vi "Sequencer Pro.vi"(8 "error in (no error)":errorcluster) -> (0 "Error State":errorcluster)   [LabVIEW 2017]
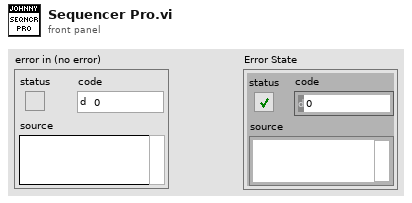
[diagram p1: front panel]
types:
  T1 = cluster{"Error State":errorcluster, "State_ndx":i32, "Timeout [s]":dbl}
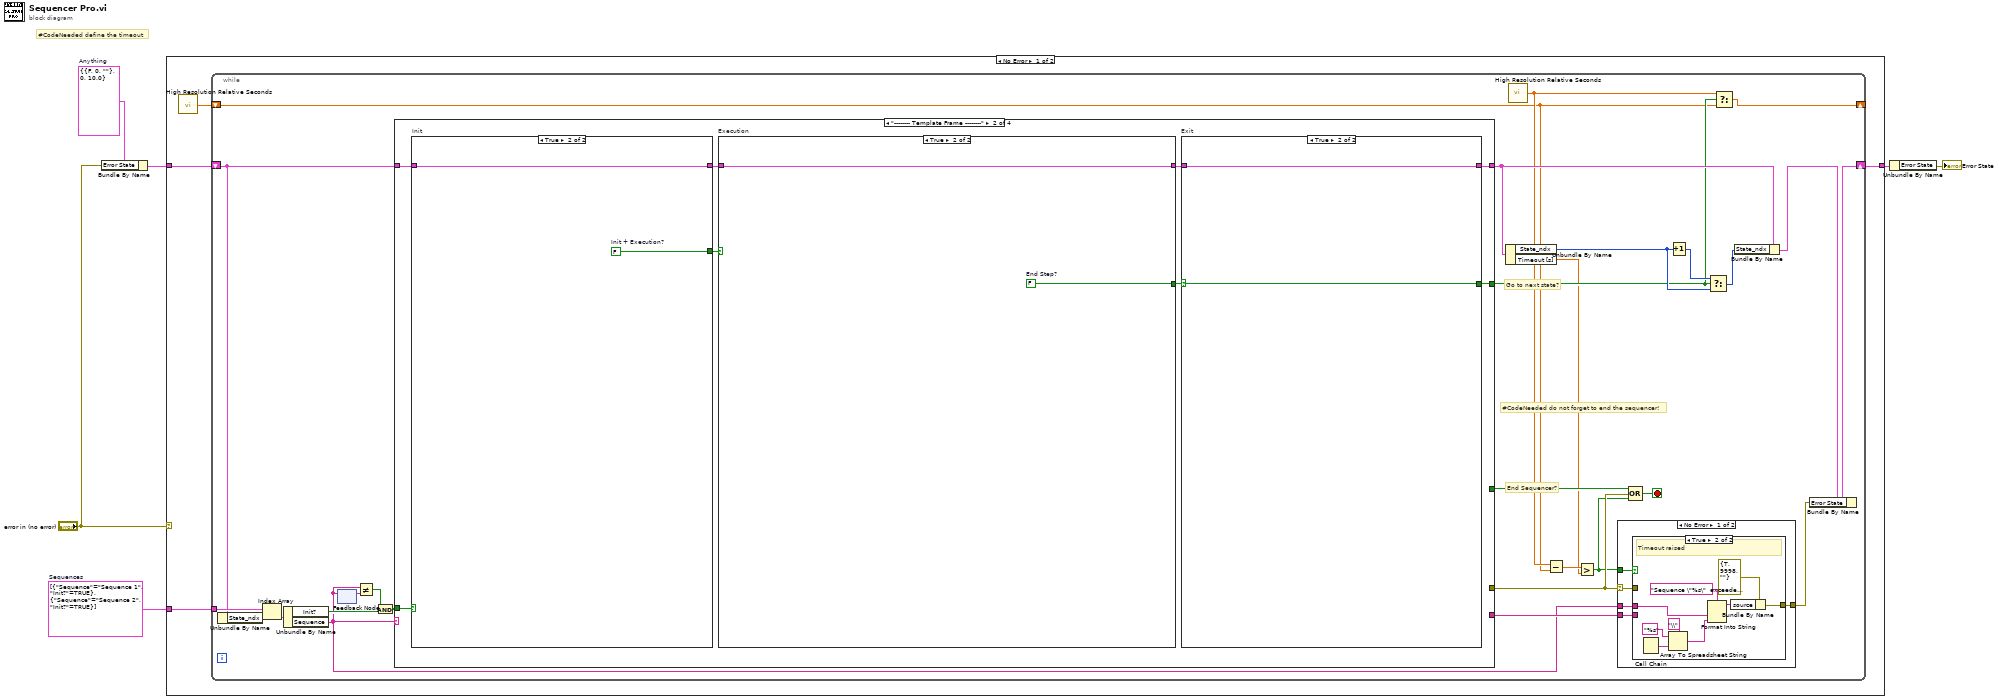
[diagram p0: block diagram]
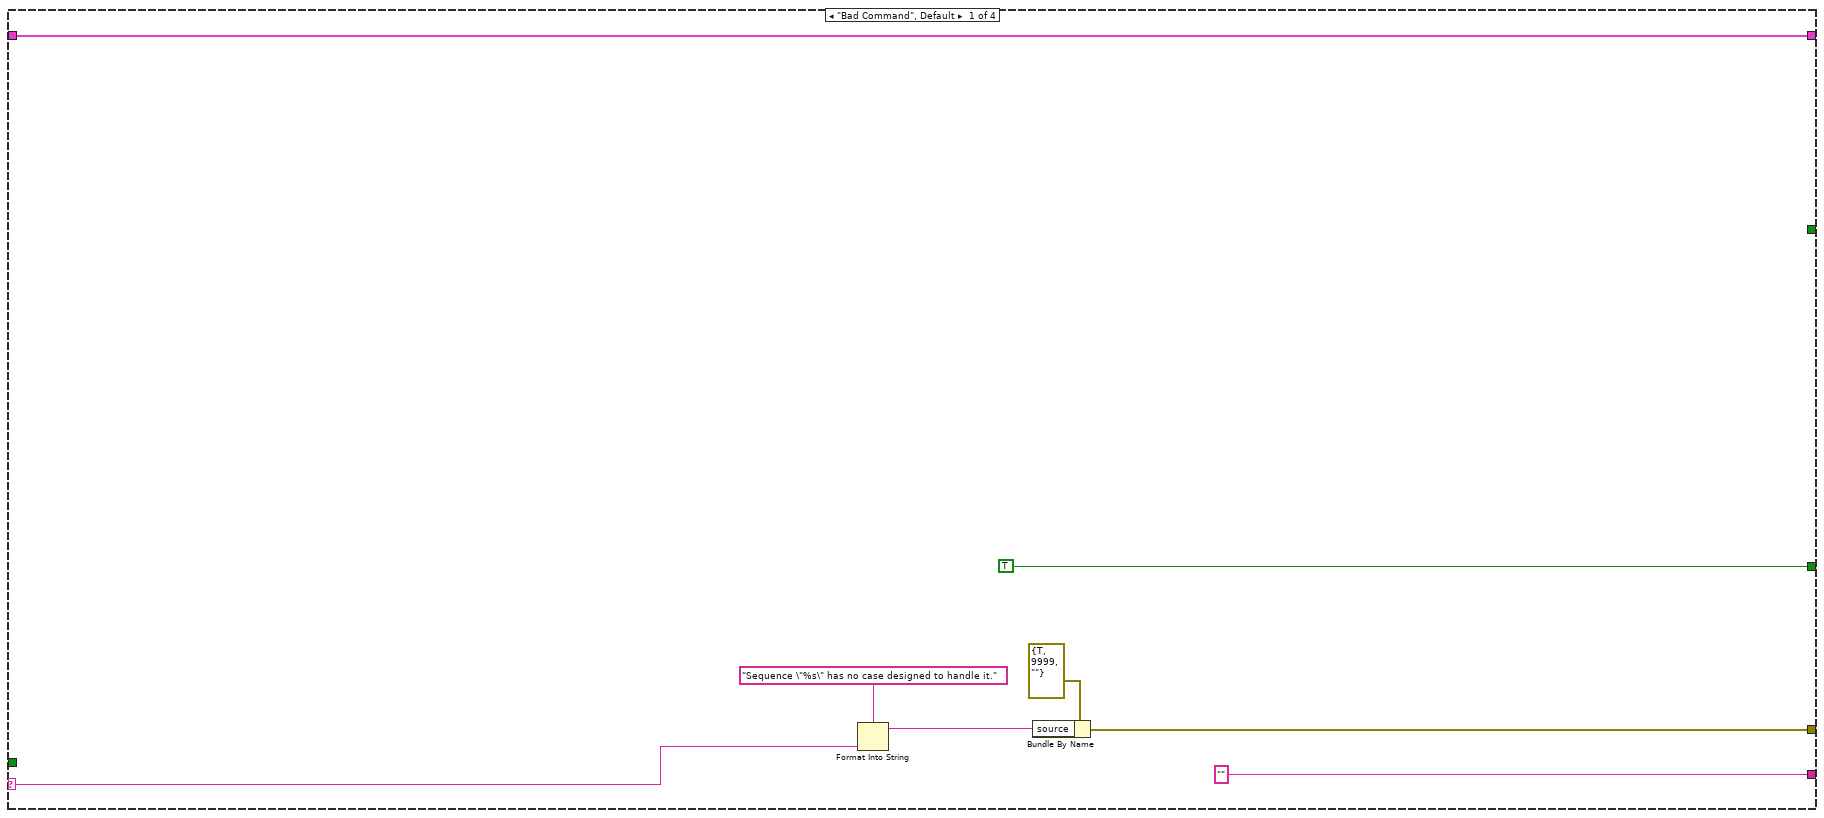
[diagram p2: hidden frame]
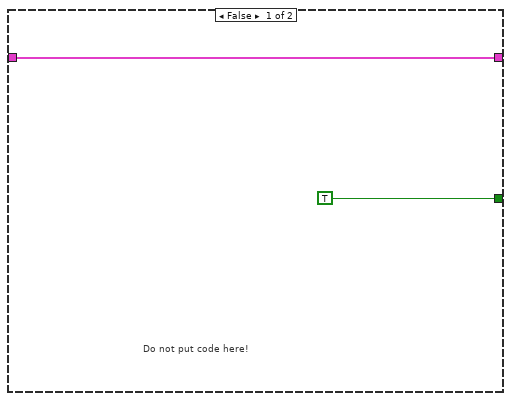
[diagram p5: hidden frame]
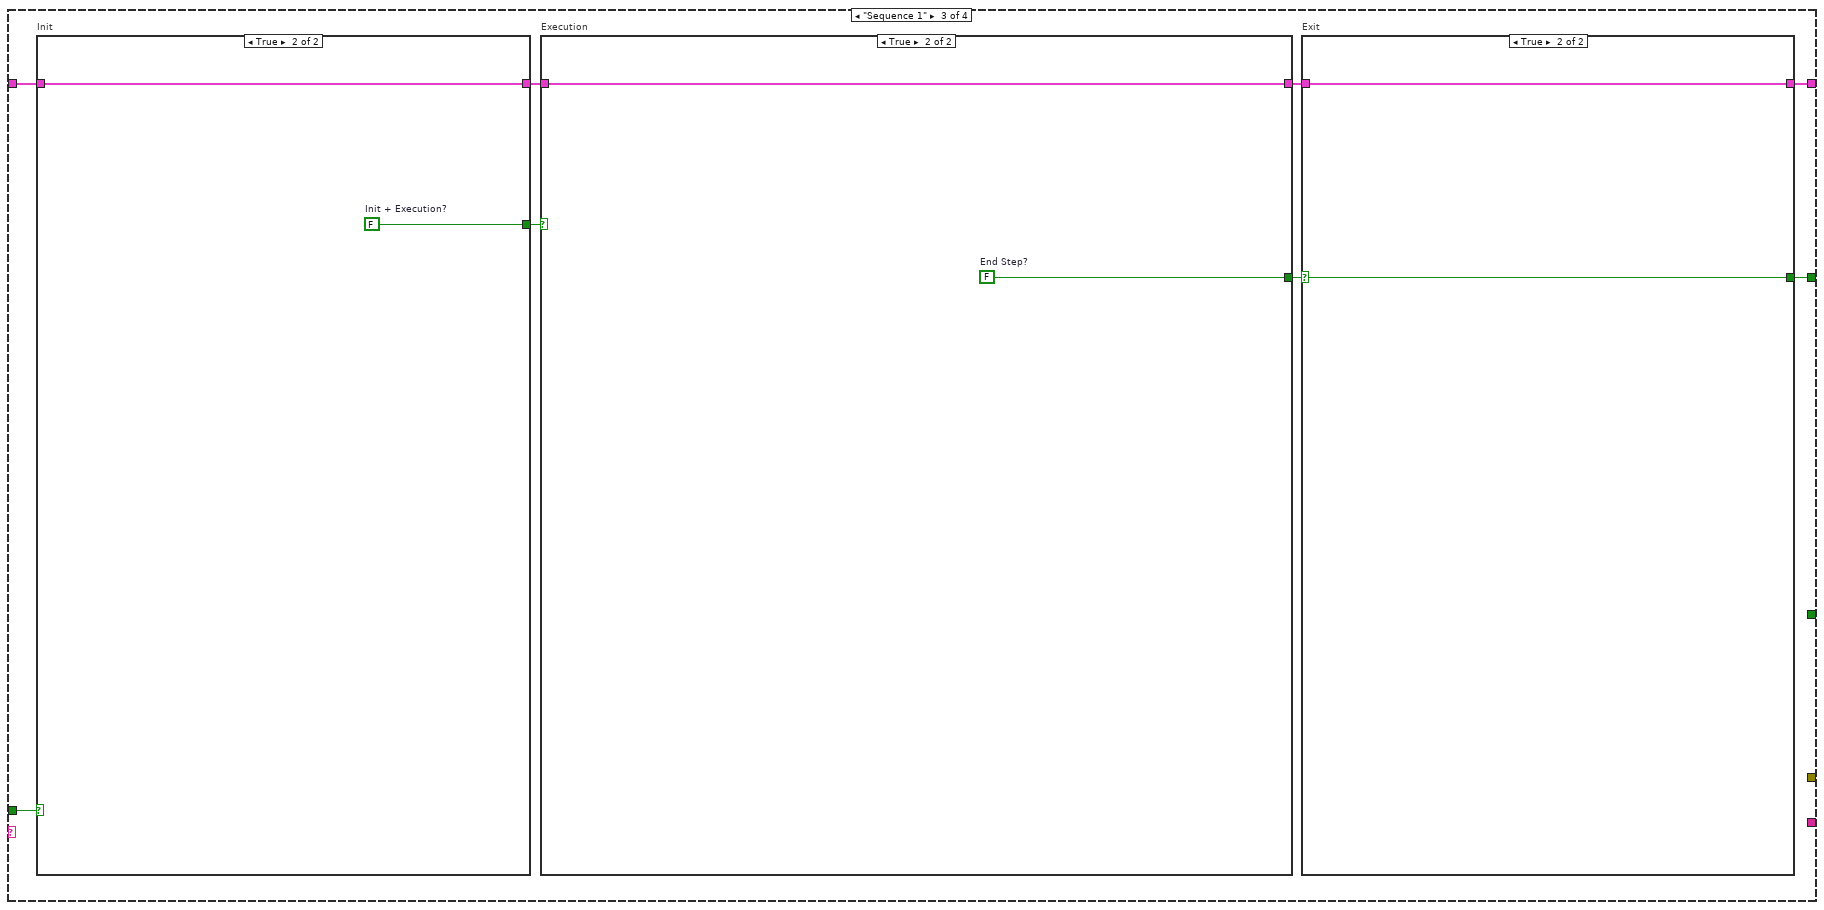
[diagram p6: hidden frame]
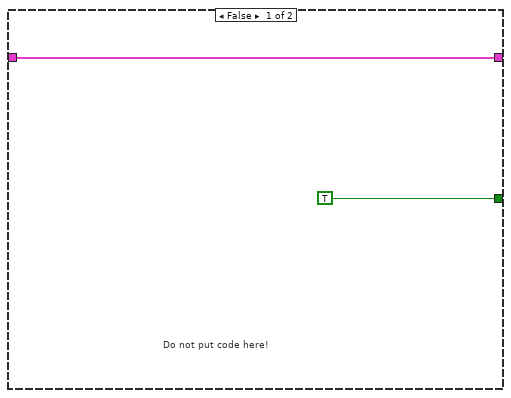
[diagram p9: hidden frame]
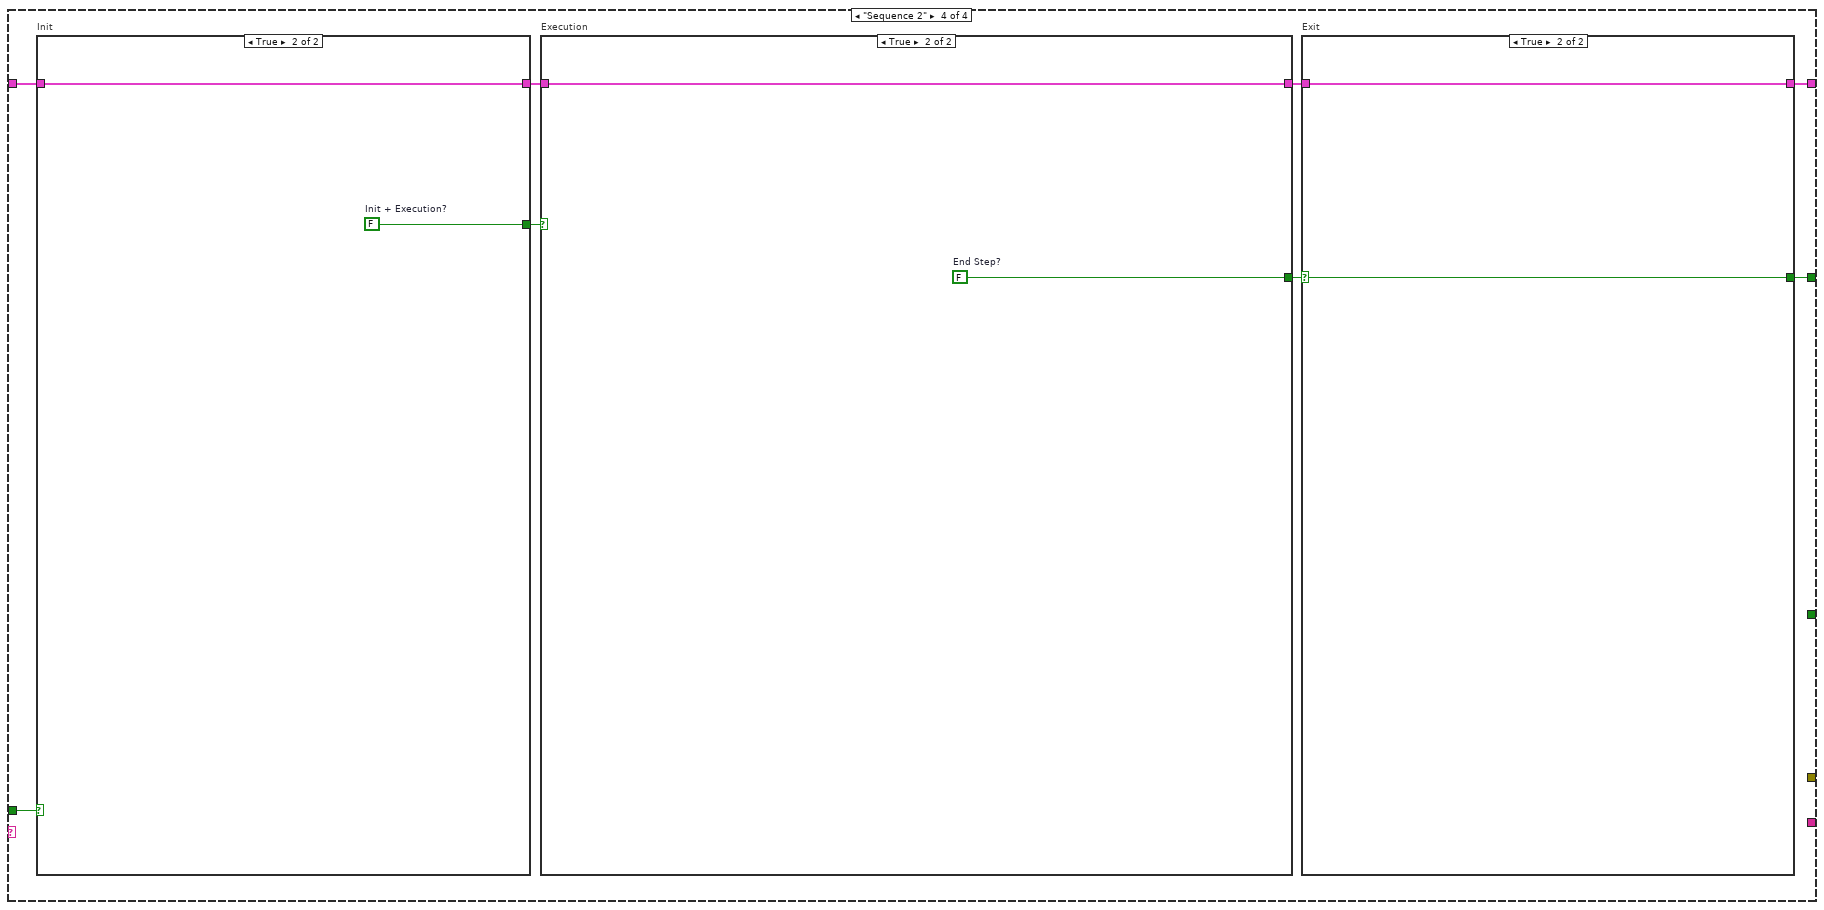
[diagram p10: hidden frame]
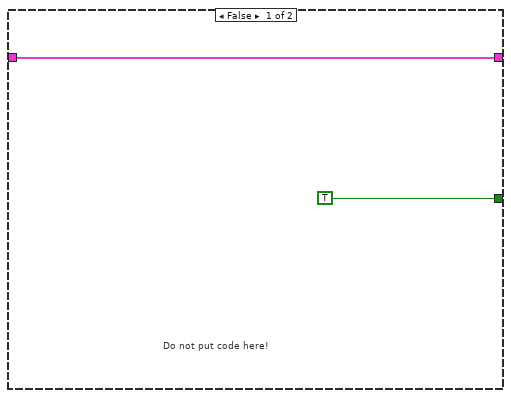
[diagram p13: hidden frame]
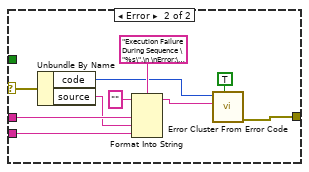
[diagram p15: hidden frame]
diagram:
  w2 = T1 {"Error State"={"status"=FALSE, "code"=0, "source"=""}, "State_ndx"=0, "Timeout [s]"=10.0}  # Anything
  w5 = cluster{"Sequence":string, "Init?":bool}[] [{"Sequence"="Sequence 1", "Init?"=TRUE}, {"Sequence"="Sequence 2", "Init?"=TRUE}]  # Sequences
  # "#CodeNeeded define the timeout"
  n1 = Bundle By Name(cluster=w2, "Error State"="error in (no error)") -> (w6:T1)
  n2 = case shown="No Error" "error in (no error)" {
    tunnel: w5 -> [w10 _]
    tunnel: w6 -> [w9 w125]
    tunnel: [w8 w125] -> w3
    frame No Error {
      n3 = call <vilib>:"High Resolution Relative Seconds.vi"() -> ("relative seconds"=w7:dbl)
      n4 = while {
        tunnel: w10 -> [w36]
        shift-right: [w37] -> w8
        shift-left: w9 -> [w33]
        shift-right: [w21] -> _
        shift-left: w7 -> [w22]
        stop <- w25 stop-if-true
        # "#CodeNeeded do not forget to end the sequencer!"
        # "End Sequencer?"
        # "Go to next state?"
        n5 = Unbundle By Name(w33) -> ("State_ndx"=w32:i32)
        n6 = Index Array(array=w36, index=w32) -> (element=w16:cluster{"Sequence":string, "Init?":bool})
        n7 = Unbundle By Name(w16) -> ("Init?"=w15:bool, "Sequence"=w14:string)
        n8 = feedback-in #1(w14) -> ()
        n9 = feedback #1() -> (w13:string)  [unwired: 1 in]
        n10 = Not Equal?(x=w14, y=w13) -> (x != y?=w11:bool)
        n11 = And(x=w11, y=w15) -> (x .and. y?=w12:bool)
        n12 = case shown="\"-------- Template Frame --------\"" w14 {
          selector: w14 -> [w40 _ _ _]
          tunnel: w33 -> [w45 w46 w64 w82]
          tunnel: [w45 w49 w67 w85] -> w30
          tunnel: [w42 _ _ _] -> w18
          tunnel: ["" ("Accessors:Name") _ _ _] -> w35
          tunnel: [_ w52 w70 w88] -> w24
          tunnel: [TRUE _ _ _] -> w26
          tunnel: w12 -> [_ w53 w71 w89]
          frame "Bad Command", Default {
            n13 = Format Into String(format string="Sequence \"%s\" has no case designed to handle it.", w40) -> (resulting string=w39:string)  [unwired: 2 in, 1 out]
            n14 = Bundle By Name(cluster=errorcluster {"status"=TRUE, "code"=9999, "source"=""} ("error out"), "source"=w39) -> (w42:errorcluster)
          }
          frame "-------- Template Frame --------" {
            n15 = case "Init" shown="True" w53 {
              tunnel: [TRUE ("Init + Execution?") w63] -> w51
              tunnel: [w60 w62] -> w47
              tunnel: w46 -> [w60 w62]
              frame False {
                # "Do not put code here!"
                # "Init"
              }
              frame True {
                w63 = FALSE  # Init + Execution?
                # "Init"
              }
            }
            n16 = case "Execution" shown="True" w51 {
              tunnel: [_ w56] -> w50
              tunnel: [w54 w55] -> w48
              tunnel: w47 -> [w54 w55]
              frame False {
                # "Do not put code here!"
                # "Execution"
              }
              frame True {
                w56 = FALSE  # End Step?
                # "Execution"
              }
            }
            n17 = case "Exit" shown="True" w50 {
              selector: w50 -> [_ w59]
              tunnel: [_ w59] -> w52
              tunnel: [w57 w58] -> w49
              tunnel: w48 -> [w57 w58]
              frame False {
                # "Do not put code here!"
                # "Exit"
              }
              frame True {
                # "Exit"
              }
            }
          }
          frame "Sequence 1" {
            n18 = case "Init" shown="True" w71 {
              tunnel: [TRUE ("Init + Execution?") w81] -> w69
              tunnel: [w78 w80] -> w65
              tunnel: w64 -> [w78 w80]
              frame False {
                # "Do not put code here!"
                # "Init"
              }
              frame True {
                w81 = FALSE  # Init + Execution?
                # "Init"
              }
            }
            n19 = case "Execution" shown="True" w69 {
              tunnel: [_ w73] -> w68
              tunnel: [w72 w74] -> w66
              tunnel: w65 -> [w72 w74]
              frame False {
                # "Do not put code here!"
                # "Execution"
              }
              frame True {
                w73 = FALSE  # End Step?
                # "Execution"
              }
            }
            n20 = case "Exit" shown="True" w68 {
              selector: w68 -> [_ w77]
              tunnel: [_ w77] -> w70
              tunnel: [w75 w76] -> w67
              tunnel: w66 -> [w75 w76]
              frame False {
                # "Do not put code here!"
                # "Exit"
              }
              frame True {
                # "Exit"
              }
            }
          }
          frame "Sequence 2" {
            n21 = case "Init" shown="True" w89 {
              tunnel: [TRUE ("Init + Execution?") w99] -> w87
              tunnel: [w96 w98] -> w83
              tunnel: w82 -> [w96 w98]
              frame False {
                # "Do not put code here!"
                # "Init"
              }
              frame True {
                w99 = FALSE  # Init + Execution?
                # "Init"
              }
            }
            n22 = case "Execution" shown="True" w87 {
              tunnel: [_ w91] -> w86
              tunnel: [w90 w92] -> w84
              tunnel: w83 -> [w90 w92]
              frame False {
                # "Do not put code here!"
                # "Execution"
              }
              frame True {
                w91 = FALSE  # End Step?
                # "Execution"
              }
            }
            n23 = case "Exit" shown="True" w86 {
              selector: w86 -> [_ w95]
              tunnel: [_ w95] -> w88
              tunnel: [w93 w94] -> w85
              tunnel: w84 -> [w93 w94]
              frame False {
                # "Do not put code here!"
                # "Exit"
              }
              frame True {
                # "Exit"
              }
            }
          }
        }
        n24 = Unbundle By Name(w30) -> ("State_ndx"=w27:i32, "Timeout [s]"=w19:dbl)
        n25 = call <vilib>:"High Resolution Relative Seconds.vi"() -> ("relative seconds"=w23:dbl)
        n26 = Subtract(x=w23, y=w22) -> (x-y=w20:dbl)
        n27 = Greater?(x=w20, y=w19) -> (0:w17:bool)
        n28 = case shown="No Error" w18 {
          selector: w18 -> [w102 w118]
          tunnel: [w103 w123] -> w34
          tunnel: w14 -> [w101 w121]
          tunnel: w35 -> [w100 w116]
          tunnel: w17 -> [w104 _]
          frame No Error {
            n29 = case shown="True" w104 {
              tunnel: w101 -> [_ w113]
              tunnel: [w105 w110] -> w103
              tunnel: w102 -> [w105 _]
              tunnel: w100 -> [_ _]
              frame False {
              }
              frame True {
                # "Timeout raised"
                n30 = Call Chain() -> (call chain=w109:string[])
                n31 = Array To Spreadsheet String(delimiter (Tab)="\\", array=w109, 3:"%s") -> (spreadsheet string=w106:string)
                n32 = Format Into String(format string="Sequence \"%s\"  exceeded the timeout.\n\n%s" ("source"), w113, w106) -> (resulting string=w111:string)  [unwired: 2 in, 1 out]
                n33 = Bundle By Name(cluster=errorcluster {"status"=TRUE, "code"=9998, "source"=""} ("error out"), "source"=w111) -> (w110:errorcluster)
              }
            }
          }
          frame Error {
            n34 = Unbundle By Name(w118) -> ("code"=w115:i32, "source"=w117:string)
            n35 = Format Into String(format string="Execution Failure During Sequence \"%s\".\n \nError:\n%s\n\n%s" ("error message (\"\")"), initial string="", w121, w117, w116) -> (resulting string=w122:string)  [unwired: 1 in, 1 out]
            n36 = call <vilib>:"Error Cluster From Error Code.vi"("show call chain? (False)"=TRUE, "error message (\"\")"=w122, "error code (0)"=w115) -> ("error out"=w123:errorcluster)  [unwired: 6 in]
          }
        }
        n37 = Compound Arithmetic op=OR(w26, w18, w17) -> (w25:bool)
        n38 = Increment(x=w27) -> (x+1=w29:i32)
        n39 = Select(t=w29, s=w24, f=w27) -> (s? t:f=w28:i32)
        n40 = Select(t=w23, s=w24, f=w22) -> (s? t:f=w21:dbl)
        n41 = Bundle By Name(cluster=w30, "State_ndx"=w28) -> (w31:T1)
        n42 = Bundle By Name(cluster=w31, "Error State"=w34) -> (w37:T1)
      }
    }
    frame Error {
    }
  }
  n43 = Unbundle By Name(w3) -> ("Error State"=→"Error State":errorcluster)
